vi "New Queue Sink.vi"(8 "error in (no error)":errorcluster, 11 "Queue Name":string) -> (0 "error out":errorcluster, 3 "Queue Sink out":refnum<class "Queue Sink.lvclass">)   [LabVIEW 2020, in "LV Log.lvlib" / "Queue Sink.lvclass"]
uses:
  Queue Sink.lvclass
  Queue Sink.lvclass/Queue Sink.ctl
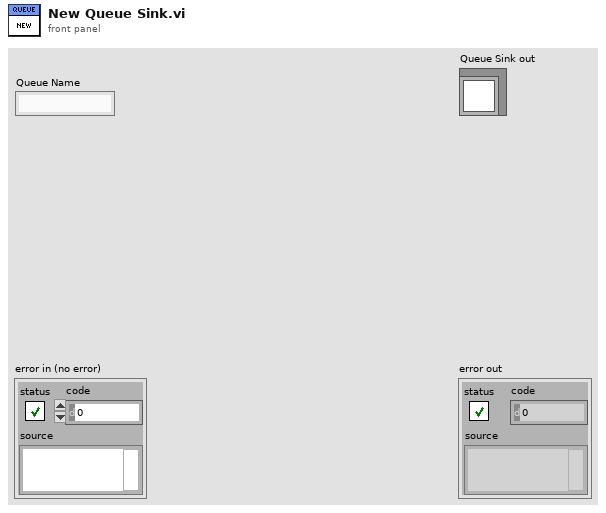
[diagram p1: front panel]
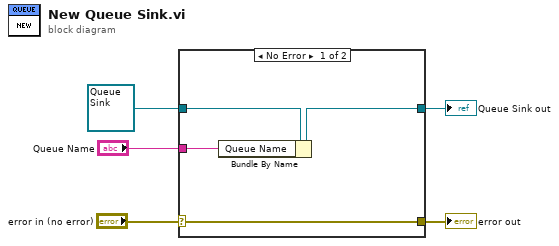
[diagram p0: block diagram]
diagram:
  n1 = case shown="No Error" "error in (no error)" {
    selector: "error in (no error)" -> [w9 w11]
    tunnel: [w9 w11] -> w4
    tunnel: [w7 w10] -> w2
    tunnel: refnum<class "Queue Sink.lvclass"> refnum ("Queue Sink in") -> [w8 w10]
    tunnel: "Queue Name" -> [w6 _]
    frame No Error {
      n2 = Bundle By Name(cluster=w8, "Queue Name"=w6) -> (w7:refnum<class "Queue Sink.lvclass">)
    }
    frame Error {
    }
  }
  "error out" <- w4
  "Queue Sink out" <- w2
